vi "Create Second Zip.vi"(3 "Status":string, 5 "Compilation Type":T1, 7 "VIPath":path caption="Deploy .vi", 8 "error in":errorcluster) -> (0 "error out":errorcluster, 2 "Second ZIP":path)   [LabVIEW 2014, in "Raspberry Pi Compatible Compiler for LabVIEW.lvlib"]
uses:
  Raspberry Pi Compatible Compiler for LabVIEW.lvlib
  Compile and Download App/Custom Controls/CompileType.ctl
  <vilib>/Utility/sysdir.llb/System Directory Type.ctl
  Compiler/RasPi Compiler.lvclass/RasPi Compiler.ctl
  Compiler/RasPi Compiler.lvclass
  RasPi_Services/Downloader/Downloader.lvclass
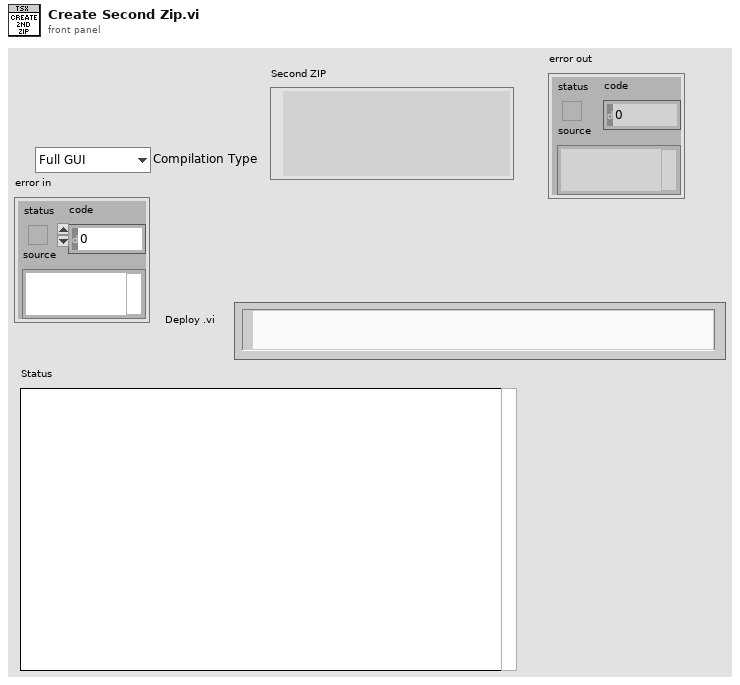
[diagram p1: front panel]
types:
  T1 = typedef "Raspberry Pi Compatible Compiler for LabVIEW.lvlib/CompileType.ctl" = enum16{"Full GUI", "Console App"}
  T2 = typedef "System Directory Type.ctl" = i32
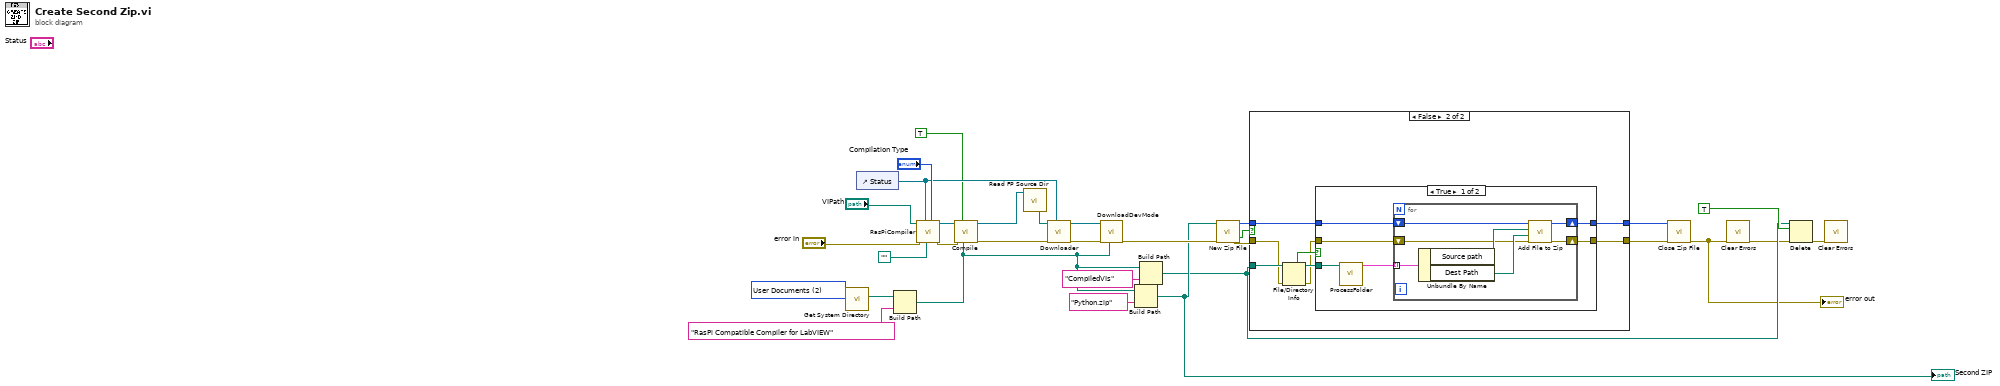
[diagram p0: block diagram]
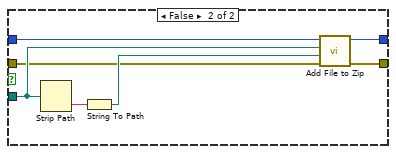
[diagram p3: hidden frame]
diagram:
  w7 = T2 2 items=["User Home"=0, "User Desktop"=1, "User Documents"=2, "User Application Data"=3, "User Preferences"=4, "User Temporary"=5, "Public Documents"=6, "Public Application Data"=7, "Public Preferences"=8, "Public Cache"=13, "System Core Libraries"=9, "System Installed Libraries"=10, "Application Files"=11, "Boot Volume Root"=12] ("system directory type")
  n1 = call <vilib>:"Get System Directory.vi"("system directory type"=w7) -> ("system directory"=w6:path)  [unwired: 10 in]
  n2 = control-ref of="Status"() -> (w24:refnum<vi>)
  n3 = Build Path(base path=w6, name or relative path="RasPi Compatible Compiler for LabVIEW") -> (appended path=w1:path)
  n4 = call "RasPiCompiler.vi"("Compilation Type"="Compilation Type", "Build Path"=path "", "Message Box"=w24, "error in"="error in", "VI Path"="VIPath") -> ("error out"=w29:errorcluster, "RasPi Compiler out"=w28:refnum<class "RasPi Compiler.lvclass">)  [unwired: 5 in]
  n5 = call "Compile.vi"("LocalCompiledDir"=w1, "DevMode"=TRUE, "error in"=w29, "RasPi Compiler in"=w28) -> ("error out"=w26:errorcluster, "RasPi Compiler out"=w27:refnum<class "RasPi Compiler.lvclass">)  [unwired: 6 in]
  n6 = call "Read FP Source Dir.vi"("RasPi Compiler in"=w27) -> ("FP Source Dir"=w25:path)  [unwired: 7 in, 1 out]
  n7 = call "Downloader.vi"("Message Box"=w24, "error in"=w26, "source"=w25) -> ("error out"=w19:errorcluster, "Downloader out"=w20:refnum<class "Downloader.lvclass">)  [unwired: 7 in]
  n8 = call "DownloadDevMode.vi"("LocalCompiledPath"=w1, "error in"=w19, "Downloader in"=w20) -> ("error out"=w18:errorcluster)  [unwired: 4 in, 2 out]
  n9 = Build Path(base path=w1, name or relative path="Python.zip") -> (appended path=w14:path)
  "Second ZIP" <- w14
  n10 = Build Path(base path=w1, name or relative path="CompiledVIs") -> (appended path=w10:path)
  n11 = call <vilib>:"New Zip File.vi"("error in (no error)"=w18, "target"=w14) -> ("error out"=w17:errorcluster, "cancelled"=w16:bool, "zip file out"=w15:i64)  [unwired: 3 in]
  n12 = case shown="False" w16 {
    tunnel: w15 -> [w33 w40]
    tunnel: w10 -> [_ w41]
    tunnel: [w33 w39] -> w9
    tunnel: w17 -> [w32 w35]
    tunnel: [w32 w38] -> w8
    frame True {
    }
    frame False {
      n13 = File/Directory Info(path=w41, error in=w35) -> (path out=w37:path, directory=w36:bool, error out=w34:errorcluster)  [unwired: 4 out]
      n14 = case shown="True" w36 {
        tunnel: w40 -> [w45 w61]
        tunnel: [w44 w60] -> w39
        tunnel: w37 -> [w47 w57]
        tunnel: w34 -> [w43 w56]
        tunnel: [w42 w55] -> w38
        frame True {
          n15 = call "ProcessFolder.vi"("Path"=w47) -> ("Array"=w46:cluster{"Source path":path, "Dest Path":path}[])  [unwired: 10 in]
          n16 = for {
            tunnel: w46 -> [w54] mode=indexing
            shift-right: [w48] -> w44
            shift-left: w45 -> [w53]
            shift-right: [w49] -> w42
            shift-left: w43 -> [w50]
            n17 = Unbundle By Name(w54) -> ("Source path"=w52:path, "Dest Path"=w51:path)
            n18 = call <vilib>:"Add File to Zip.vi"("error in (no error)"=w50, "destination path in zip"=w51, "source file path"=w52, "zip file in"=w53) -> ("error out"=w49:errorcluster, "zip file out"=w48:i64)  [unwired: 6 in]
          }
        }
        frame False {
          n19 = Strip Path(path=w57) -> (name=w59:string)  [unwired: 1 out]
          n20 = String To Path(string=w59) -> (path=w58:path)
          n21 = call <vilib>:"Add File to Zip.vi"("error in (no error)"=w56, "destination path in zip"=w58, "source file path"=w57, "zip file in"=w61) -> ("error out"=w55:errorcluster, "zip file out"=w60:i64)  [unwired: 6 in]
        }
      }
    }
  }
  n22 = call <vilib>:"Close Zip File.vi"("error in (no error)"=w8, "zip file in"=w9) -> ("error out"=w3:errorcluster)  [unwired: 5 in]
  "error out" <- w3
  n23 = call <vilib>:"Clear Errors.vi"("error in (no error)"=w3) -> ("error out"=w4:errorcluster)  [unwired: 5 in, 1 out]
  n24 = Delete(path (use dialog)=w10, entire hierarchy (F)=TRUE, error in=w4) -> (error out=w2:errorcluster)  [unwired: 2 in, 2 out]
  n25 = call <vilib>:"Clear Errors.vi"("error in (no error)"=w2) -> ()  [unwired: 5 in, 2 out]
